vi "读取数据状态.vi"(8 "error in (no error)":errorcluster) -> (0 "error out":errorcluster, 3 "簇":T1)   [LabVIEW 2016, in "一代CodMn.lvlib"]
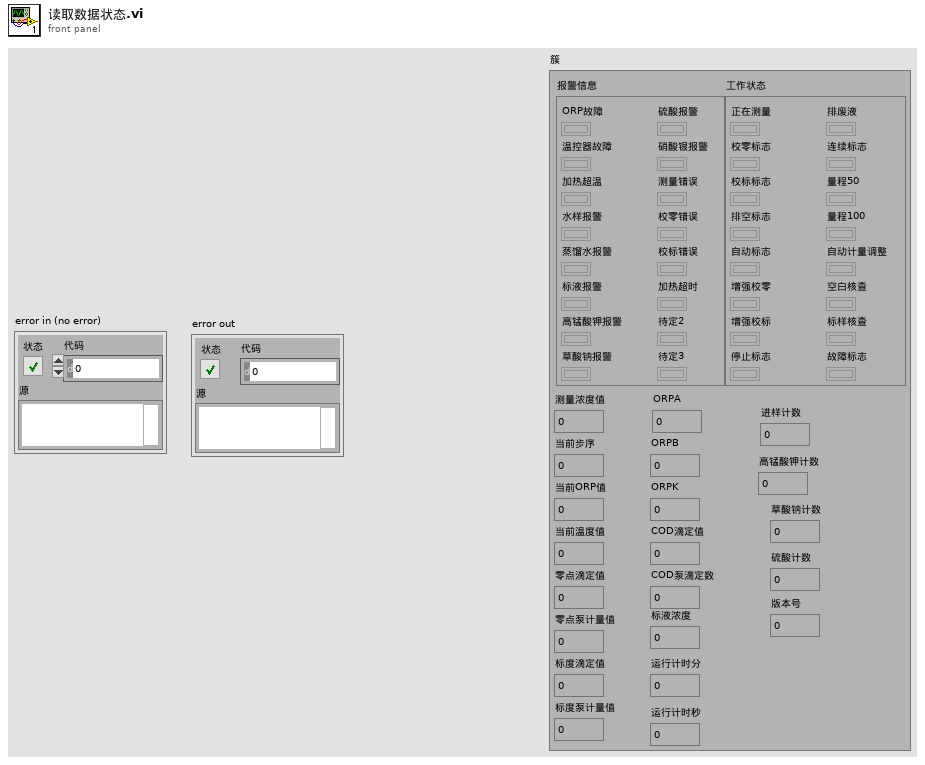
[diagram p1: front panel]
types:
  T1 = cluster{"报警信息":cluster{"ORP故障":bool, "温控器故障":bool, "加热超温":bool, "水样报警":bool, "蒸馏水报警":bool, "标液报警":bool, "高锰酸钾报警":bool, "草酸钠报警":bool, "硫酸报警":bool, "硝酸银报警":bool, "测量错误":bool, "校零错误":bool, "校标错误":bool, "加热超时":bool, "待定2":bool, "待定3":bool}, "工作状态":cluster{"正在测量":bool, "校零标志":bool, "校标标志":bool, "排空标志":bool, "自动标志":bool, "增强校零":bool, "增强校标":bool, "停止标志":bool, "排废液":bool, "连续标志":bool, "量程50":bool, "量程100":bool, "自动计量调整":bool, "空白核查":bool, "标样核查":bool, "故障标志":bool}, "测量浓度值":sgl, "当前步序":u16, "当前ORP值":i16, "当前温度值":sgl, "零点滴定值":sgl, "零点泵计量值":i16, "标度滴定值":sgl, "标度泵计量值":i16, "ORPA":i16, "ORPB":i16, "ORPK":i16, "COD滴定值":sgl, "COD泵滴定数":u16, "标液浓度":sgl, "运行计时分":u16, "运行计时秒":u16, "进样计数":u16, "高锰酸钾计数":u16, "草酸钠计数":u16, "硫酸计数":u16, "版本号":u32}
  T2 = enum16{"open", "close", "readHR", "writeHR", "readCoil", "writeCoil"}
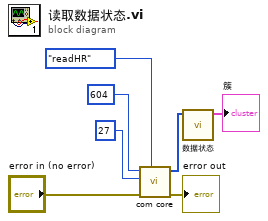
[diagram p0: block diagram]
diagram:
  n1 = call "com core.vi"("功能"=T2."readHR", "error in (no error)"="error in (no error)", "quantity"=u16 27, "starting address"=u16 604) -> ("error out"=→"error out":errorcluster, "Registers"=w7:u16[])  [unwired: 5 in, 1 out]
  n2 = call "数据状态.vi"("数组"=w7) -> ("簇"=→"簇":T1)  [unwired: 10 in]
